vi "ReceiveData.vi"(8 "error in (no error)":errorcluster, 10 "Delay before read (ms)":u32=100, 11 "VISA resource name":refnum<visa-resource-name>) -> (0 "error out":errorcluster, 1 "Raw Response":string, 2 "Recieved Data":T1, 3 "VISA resource name out":refnum<visa-resource-name>, 4 "return count":u32)   [LabVIEW 2020, in "driver_flodx_ph_probe.lvlib"]
uses:
  <instrlib>/RxnRover/FloDx Ph Probe Driver/driver_flodx_ph_probe.lvlib
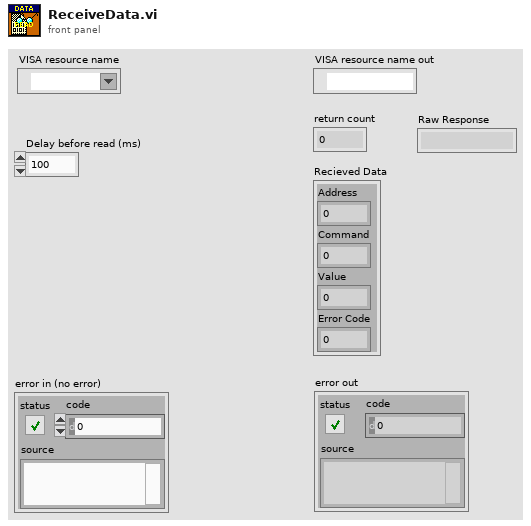
[diagram p1: front panel]
types:
  T1 = cluster{"Address":u32, "Command":u32, "Value":dbl, "Error Code":u32}
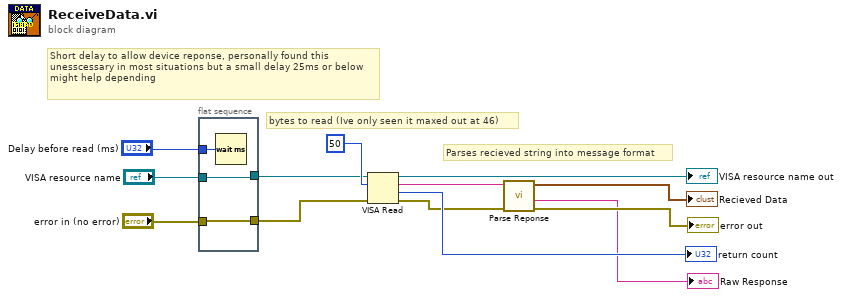
[diagram p0: block diagram]
diagram:
  # "bytes to read (Ive only seen it maxed out at 46)"
  # "Short delay to allow device reponse, personally found this unesscessary in most situations but a small delay 25ms or below might help depending"
  # "Parses recieved string into message format"
  n1 = flat-sequence {
    tunnel: "error in (no error)" -> [w15]
    tunnel: [w15] -> w3
    tunnel: [w16] -> w2
    tunnel: "VISA resource name" -> [w16]
    tunnel: "Delay before read (ms)" -> [w14]
    frame #0 {
      n2 = Wait (ms)(milliseconds to wait=w14) -> ()  [unwired: 1 out]
    }
  }
  n3 = VISA Read(VISA resource name=w2, byte count=u32 50, error in (no error)=w3) -> (VISA resource name out=→"VISA resource name out":refnum<visa-resource-name>, read buffer=w11:string, return count=→"return count":u32, error out=w10:errorcluster)
  n4 = call <instrlib>:"Parse Reponse.vi"("error in"=w10, "Input String"=w11) -> ("error out"=→"error out":errorcluster, "Raw Response"=→"Raw Response":string, "Parsed Response"=→"Recieved Data":T1)  [unwired: 7 in]
